vi "Get Limit String Length.vi"(4 "error in (no error)":errorcluster caption="错误输入（无错误）", 6 "Container State":T3 caption="容器状态", 7 "Display State In":T1={"字符串长度"=10, "过滤字符"=[8, 127], "文本字体"={"Font Name"="", "Size"=0, "Bold"=FALSE, "Italic"=FALSE, "Underline"=FALSE, "Strikeout"=FALSE, "Color"=0}} caption="显示状态输入") -> (0 "error out":errorcluster caption="错误输出", 2 "Value":u8 caption="值", 3 "Display State Out":T1={"字符串长度"=10, "过滤字符"=[8, 127], "文本字体"={"Font Name"="", "Size"=0, "Bold"=FALSE, "Italic"=FALSE, "Underline"=FALSE, "Strikeout"=FALSE, "Color"=0}} caption="显示状态输出")   [LabVIEW 2013, in "Limit String.xctl"]
uses:
  Limit String.xctl
  <vilib>/_xctls/Container State.ctl
  <vilib>/Utility/miscctls.llb/LVFontTypeDef.ctl
  <vilib>/_xctls/XControlSupport.lvlib
panel:
  # "将以下值显示控件替换为所需类型的显示控件。\n不要从连线板中删除该显示控件或其它显示控件。\n不要更改连线板模式。\n值显示控件应始终位于连线板输出端自顶部起第二个接线端。"
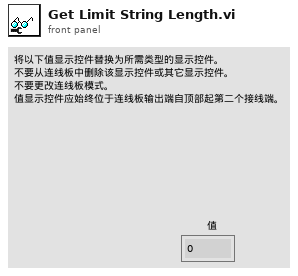
[diagram p1: front panel]
types:
  T1 = typedef "Limit String.xctl/状态.ctl" = cluster{"字符串长度":u8, "过滤字符":i16[], "文本字体":T2}
  T2 = typedef "LVFontTypeDef.ctl" = cluster{"Font Name":string, "Size":u16, "Bold":bool, "Italic":bool, "Underline":bool, "Strikeout":bool, "Color":u32}
  T3 = typedef "XControlSupport.lvlib/Container State.ctl" = cluster{"Indicator?":bool, "Run Mode?":bool, " Refnum":refnum<vi>}
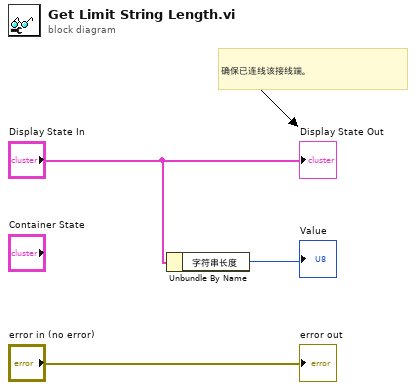
[diagram p0: block diagram]
diagram:
  # "确保已连线该接线端。"
  n1 = Unbundle By Name("Display State In") -> ("字符串长度"=→"Value":u8)
  "error out" <- "error in (no error)"
  "Display State Out" <- "Display State In"
